vi "Data Parameters FG.vi"(7 "Action":T1, 8 "error in (no error)":errorcluster, 10 "Data Parameters":T3={"Data Type"=enum."Single Channel", "Channel Type"=enum."Format", "Format String"="%.3g", "Expected String"="", "Type"=enum."SGL", "List"=[], "Delimiter"=",", "Endian"=enum."Native"}, 11 "Item Ref in":T2 format="%.0x") -> (0 "error out":errorcluster, 2 "Data Parameters":T3={"Data Type"=enum."Single Channel", "Channel Type"=enum."Format", "Format String"="%.3g", "Expected String"="", "Type"=enum."SGL", "List"=[], "Delimiter"=",", "Endian"=enum."Native"}, 3 "Item Ref out":T2 format="%.0x")   [LabVIEW 2020, in "Instrument Addon Shared.lvlib"]
uses:
  Instrument Addon Shared.lvlib
  Data Parameters.ctl
  Protocol Data Type.ctl
  Data Channel Type.ctl
  Type Cast Type.ctl
  Endian.ctl
  <vilib>/NI VeriStand/Custom Device API/Custom Device Item Ref.ctl
  FG Control.ctl
  Constants.vi
  <vilib>/NI VeriStand/Custom Device API/Get Item Property (U32).vi
  <vilib>/NI VeriStand/Custom Device API/Get Item Property (String).vi
  <vilib>/NI VeriStand/Custom Device API/Get Item Property (String Array).vi
  <vilib>/NI VeriStand/Custom Device API/Set Item Property (U32).vi
  <vilib>/NI VeriStand/Custom Device API/Set Item Property (String).vi
  <vilib>/NI VeriStand/Custom Device API/Set Item Property (String Array).vi
  <vilib>/NI VeriStand/Custom Device API/Custom Device API.lvlib
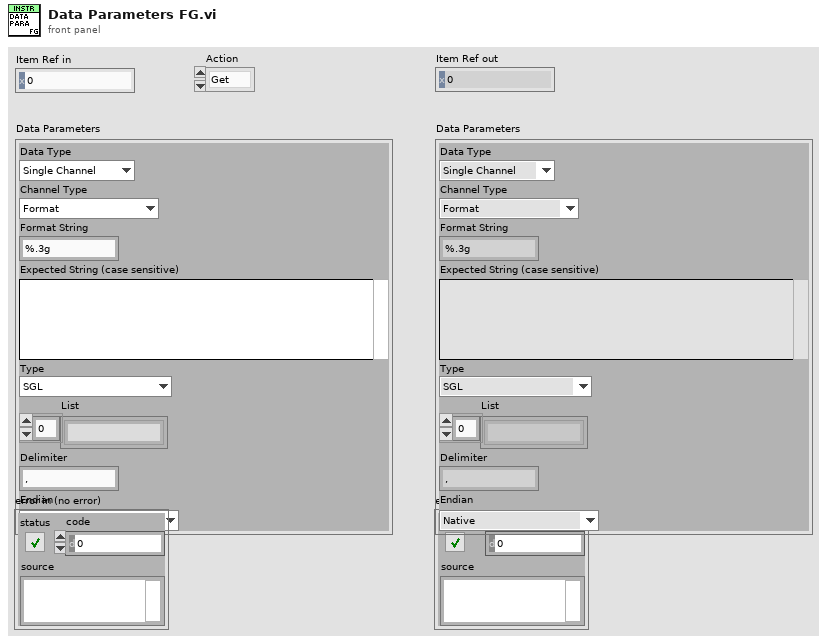
[diagram p1: front panel]
types:
  T1 = typedef "Instrument Addon Shared.lvlib/FG Control.ctl" = enum16{"Get", "Set"}
  T2 = typedef "Custom Device API.lvlib/Custom Device Item Ref.ctl" = u64
  T3 = typedef "Instrument Addon Shared.lvlib/Data Parameters.ctl" = cluster{"Data Type":T4, "Channel Type":T5, "Format String":string, "Expected String":string, "Type":T6, "List":string[], "Delimiter":string, "Endian":T7}
  T4 = typedef "Instrument Addon Shared.lvlib/Protocol Data Type.ctl" = enum16{"Single Channel", "Array"}
  T5 = typedef "Instrument Addon Shared.lvlib/Data Channel Type.ctl" = enum16{"Format", "Comparison", "Type Cast", "Enumerated List"}
  T6 = typedef "Instrument Addon Shared.lvlib/Type Cast Type.ctl" = enum16{"DBL", "SGL", "U64", "U32", "U16", "U8", "I64", "I32", "I16", "I8"}
  T7 = typedef "Instrument Addon Shared.lvlib/Endian.ctl" = enum16{"Native", "Little", "Big"}
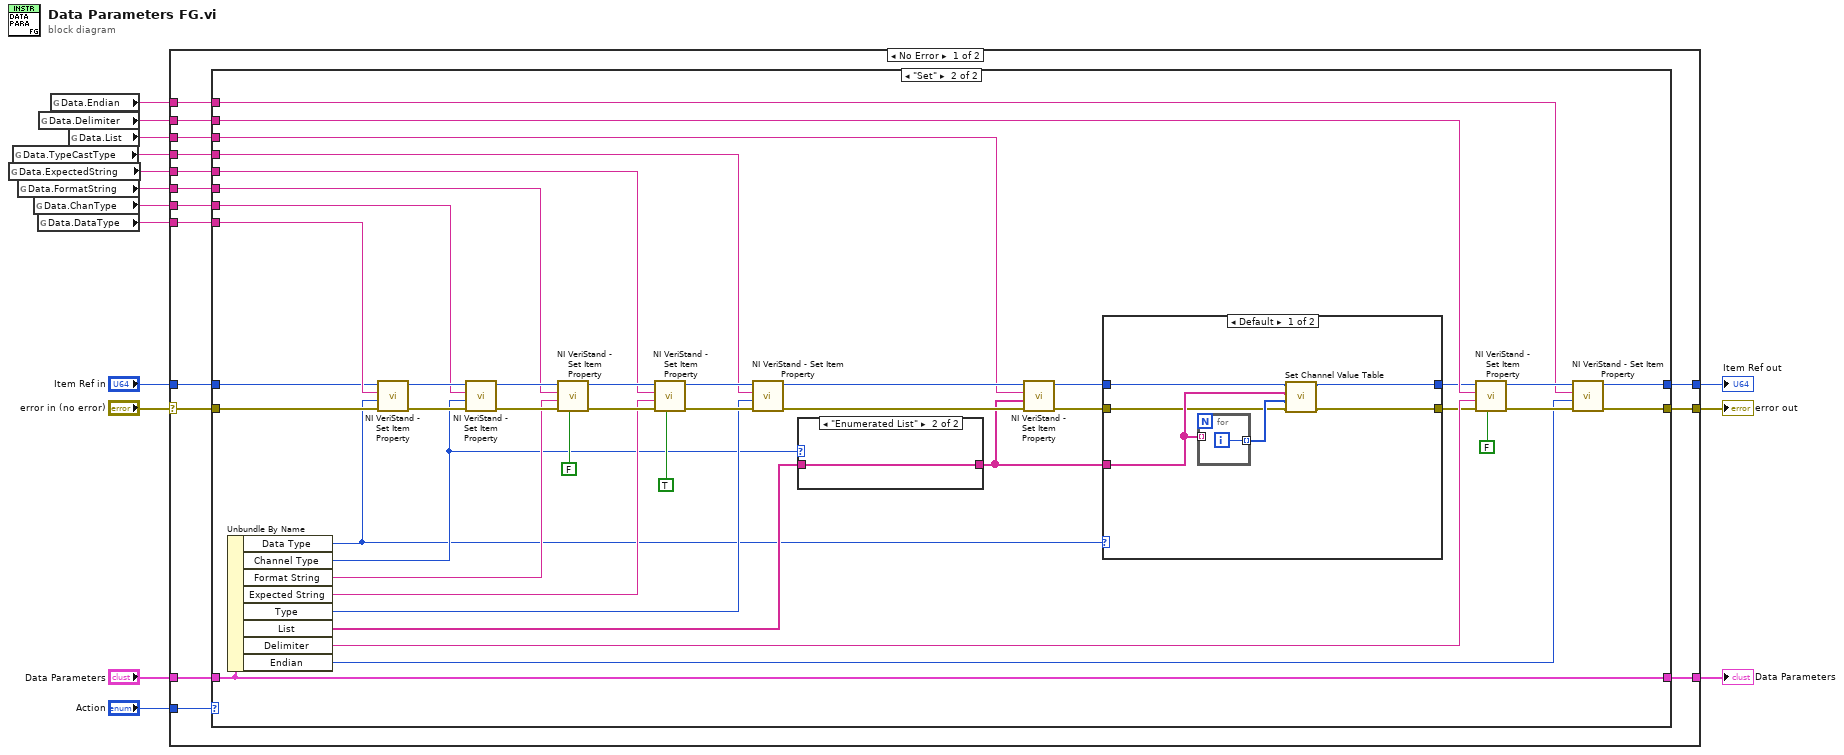
[diagram p0: block diagram]
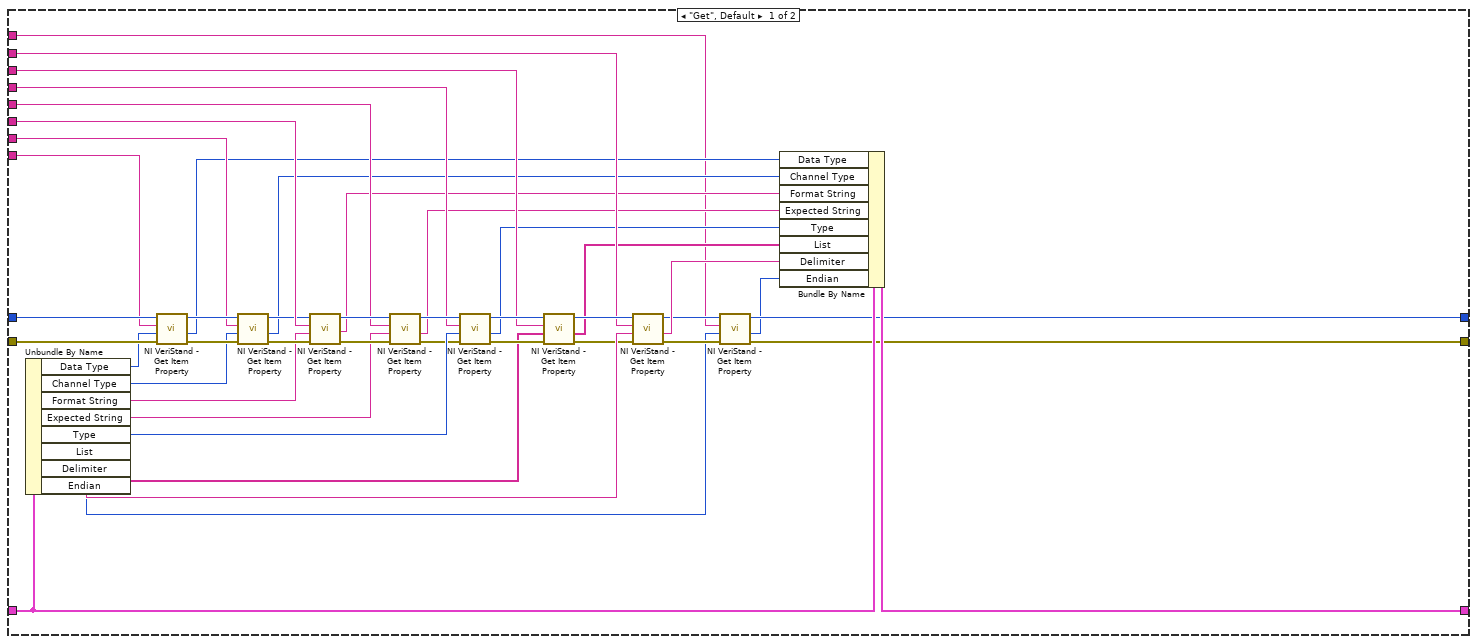
[diagram p2: hidden frame]
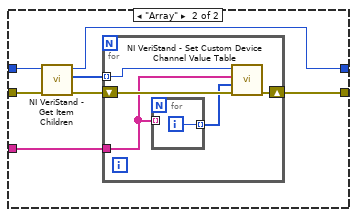
[diagram p3: hidden frame]
diagram:
  n1 = global read "Constants.vi" "Data.ExpectedString"() -> (w5:string)
  n2 = global read "Constants.vi" "Data.TypeCastType"() -> (w4:string)
  n3 = global read "Constants.vi" "Data.FormatString"() -> (w6:string)
  n4 = global read "Constants.vi" "Data.ChanType"() -> (w7:string)
  n5 = global read "Constants.vi" "Data.DataType"() -> (w9:string)
  n6 = global read "Constants.vi" "Data.Delimiter"() -> (w2:string)
  n7 = global read "Constants.vi" "Data.Endian"() -> (w1:string)
  n8 = global read "Constants.vi" "Data.List"() -> (w3:string)
  n9 = case shown="No Error" "error in (no error)" {
    selector: "error in (no error)" -> [w25 w139]
    tunnel: w9 -> [w30 _]
    tunnel: [w29 w137] -> w13
    tunnel: "Item Ref in" -> [w28 w137]
    tunnel: "Data Parameters" -> [w27 w138]
    tunnel: [w26 w139] -> w12
    tunnel: [w24 w138] -> w8
    tunnel: "Action" -> [w23 _]
    tunnel: w7 -> [w22 _]
    tunnel: w6 -> [w21 _]
    tunnel: w5 -> [w20 _]
    tunnel: w4 -> [w19 _]
    tunnel: w3 -> [w18 _]
    tunnel: w2 -> [w17 _]
    tunnel: w1 -> [w16 _]
    frame No Error {
      n10 = case shown="\"Set\"" w23 {
        tunnel: w30 -> [w72 w115]
        tunnel: [w34 w87] -> w29
        tunnel: w28 -> [w73 w114]
        tunnel: w27 -> [w46 w112]
        tunnel: [w35 w88] -> w26
        tunnel: w25 -> [w74 w113]
        tunnel: [w45 w112] -> w24
        tunnel: w22 -> [w67 w96]
        tunnel: w21 -> [w66 w95]
        tunnel: w20 -> [w50 w94]
        tunnel: w19 -> [w49 w93]
        tunnel: w18 -> [w48 w92]
        tunnel: w17 -> [w47 w91]
        tunnel: w16 -> [w32 w86]
        frame "Get", Default {
          n11 = Unbundle By Name(w46) -> ("Data Type"=w71:T4, "Channel Type"=w68:T5, "Format String"=w63:string, "Expected String"=w60:string, "Type"=w59:T6, "List"=w55:string[], "Delimiter"=w54:string, "Endian"=w33:T7)
          n12 = call-poly <vilib>:"NI VeriStand - Get Item Property.vi"("error in (no error)"=w74, "Default Value"=w71, "Property Name"=w72, "Item Ref in"=w73) -> ("error out"=w69:errorcluster, "Value"=w38:u32, "Item Ref out"=w70:T2)  [unwired: 4 in, 1 out]
          n13 = call-poly <vilib>:"NI VeriStand - Get Item Property.vi"("error in (no error)"=w69, "Default Value"=w68, "Property Name"=w67, "Item Ref in"=w70) -> ("error out"=w64:errorcluster, "Value"=w39:u32, "Item Ref out"=w65:T2)  [unwired: 4 in, 1 out]
          n14 = call-poly <vilib>:"NI VeriStand - Get Item Property.vi"("error in (no error)"=w64, "Default Value"=w63, "Property Name"=w66, "Item Ref in"=w65) -> ("error out"=w61:errorcluster, "Value"=w40:string, "Item Ref out"=w62:T2)  [unwired: 4 in, 1 out]
          n15 = call-poly <vilib>:"NI VeriStand - Get Item Property.vi"("error in (no error)"=w61, "Default Value"=w60, "Property Name"=w50, "Item Ref in"=w62) -> ("error out"=w58:errorcluster, "Value"=w41:string, "Item Ref out"=w57:T2)  [unwired: 4 in, 1 out]
          n16 = call-poly <vilib>:"NI VeriStand - Get Item Property.vi"("error in (no error)"=w58, "Default Value"=w59, "Property Name"=w49, "Item Ref in"=w57) -> ("error out"=w56:errorcluster, "Value"=w42:u32, "Item Ref out"=w52:T2)  [unwired: 4 in, 1 out]
          n17 = call-poly <vilib>:"NI VeriStand - Get Item Property.vi"("error in (no error)"=w56, "Default Value"=w55, "Property Name"=w48, "Item Ref in"=w52) -> ("error out"=w53:errorcluster, "Value"=w43:string[], "Item Ref out"=w51:T2)  [unwired: 4 in, 1 out]
          n18 = call-poly <vilib>:"NI VeriStand - Get Item Property.vi"("error in (no error)"=w53, "Default Value"=w54, "Property Name"=w47, "Item Ref in"=w51) -> ("error out"=w36:errorcluster, "Value"=w44:string, "Item Ref out"=w37:T2)  [unwired: 4 in, 1 out]
          n19 = call-poly <vilib>:"NI VeriStand - Get Item Property.vi"("error in (no error)"=w36, "Default Value"=w33, "Property Name"=w32, "Item Ref in"=w37) -> ("error out"=w35:errorcluster, "Value"=w31:u32, "Item Ref out"=w34:T2)  [unwired: 4 in, 1 out]
          n20 = Bundle By Name(cluster=w46, "Data Type"=w38, "Channel Type"=w39, "Format String"=w40, "Expected String"=w41, "Type"=w42, "List"=w43, "Delimiter"=w44, "Endian"=w31) -> (w45:T3)
        }
        frame "Set" {
          n21 = Unbundle By Name(w112) -> ("Data Type"=w75:T4, "Channel Type"=w79:T5, "Format String"=w101:string, "Expected String"=w99:string, "Type"=w98:T6, "List"=w77:string[], "Delimiter"=w97:string, "Endian"=w85:T7)
          n22 = call-poly <vilib>:"NI VeriStand - Set Item Property.vi"("error in (no error)"=w113, "Value"=w75, "Property Name"=w115, "Item Ref in"=w114) -> ("error out"=w110:errorcluster, "Item Ref out"=w111:T2)  [unwired: 5 in, 1 out]
          n23 = call-poly <vilib>:"NI VeriStand - Set Item Property.vi"("error in (no error)"=w110, "Value"=w79, "Property Name"=w96, "Item Ref in"=w111) -> ("error out"=w108:errorcluster, "Item Ref out"=w109:T2)  [unwired: 5 in, 1 out]
          n24 = call-poly <vilib>:"NI VeriStand - Set Item Property.vi"("Binary String (T)"=FALSE, "error in (no error)"=w108, "Value"=w101, "Property Name"=w95, "Item Ref in"=w109) -> ("error out"=w106:errorcluster, "Item Ref out"=w107:T2)  [unwired: 4 in, 1 out]
          n25 = call-poly <vilib>:"NI VeriStand - Set Item Property.vi"("Binary String (T)"=TRUE, "error in (no error)"=w106, "Value"=w99, "Property Name"=w94, "Item Ref in"=w107) -> ("error out"=w104:errorcluster, "Item Ref out"=w105:T2)  [unwired: 4 in, 1 out]
          n26 = call-poly <vilib>:"NI VeriStand - Set Item Property.vi"("error in (no error)"=w104, "Value"=w98, "Property Name"=w93, "Item Ref in"=w105) -> ("error out"=w103:errorcluster, "Item Ref out"=w102:T2)  [unwired: 5 in, 1 out]
          n27 = case shown="\"Enumerated List\"" w79 {
            tunnel: w77 -> [_ w136]
            tunnel: [_ w136] -> w76
            frame Default {
            }
            frame "Enumerated List" {
            }
          }
          n28 = call-poly <vilib>:"NI VeriStand - Set Item Property.vi"("error in (no error)"=w103, "Value"=w76, "Property Name"=w92, "Item Ref in"=w102) -> ("error out"=w82:errorcluster, "Item Ref out"=w83:T2)  [unwired: 5 in, 1 out]
          n29 = case shown="Default" w75 {
            tunnel: w83 -> [w119 w125]
            tunnel: w82 -> [w116 w127]
            tunnel: [w120 w123] -> w81
            tunnel: [w121 w129] -> w80
            tunnel: w76 -> [w118 w128]
            frame Default {
              n30 = for {
                tunnel: w118 -> [_] mode=indexing
                tunnel: [w122] -> w117 mode=indexing
                i -> [w122]
              }
              n31 = call "Set Channel Value Table.vi"("Error In"=w116, "Values"=w117, "Names"=w118, "Channel Ref In"=w119) -> ("Error Out"=w121:errorcluster, "Channel Ref Out"=w120:T2)  [unwired: 6 in]
            }
            frame "Array" {
              n32 = call <vilib>:"NI VeriStand - Get Item Children.vi"("error in (no error)"=w127, "Item Ref in"=w125) -> ("error out"=w126:errorcluster, "Child Refs"=w124:T2[], "Item Ref out"=w123:T2)  [unwired: 6 in, 1 out]
              n33 = for {
                tunnel: w128 -> [w131]
                shift-right: [w133] -> w129
                shift-left: w126 -> [w134]
                tunnel: w124 -> [w130] mode=indexing
                n34 = for {
                  tunnel: w131 -> [_] mode=indexing
                  tunnel: [w135] -> w132 mode=indexing
                  i -> [w135]
                }
                n35 = call <vilib>:"NI VeriStand - Set Custom Device Channel Value Table.vi"("error in (no error)"=w134, "Values"=w132, "Names"=w131, "Channel Ref in"=w130) -> ("error out"=w133:errorcluster)  [unwired: 6 in, 1 out]
              }
            }
          }
          n36 = call-poly <vilib>:"NI VeriStand - Set Item Property.vi"("Binary String (T)"=FALSE, "error in (no error)"=w80, "Value"=w97, "Property Name"=w91, "Item Ref in"=w81) -> ("error out"=w89:errorcluster, "Item Ref out"=w90:T2)  [unwired: 4 in, 1 out]
          n37 = call-poly <vilib>:"NI VeriStand - Set Item Property.vi"("error in (no error)"=w89, "Value"=w85, "Property Name"=w86, "Item Ref in"=w90) -> ("error out"=w88:errorcluster, "Item Ref out"=w87:T2)  [unwired: 5 in, 1 out]
        }
      }
    }
    frame Error {
    }
  }
  "error out" <- w12
  "Data Parameters" <- w8
  "Item Ref out" <- w13
